vi "Img Update Basic Point.vi"(8 "error in (no error)":errorcluster, 11 "LF2R IDE in":refnum<class "Main Panel.lvclass">) -> (0 "error out":errorcluster, 3 "LF2R IDE out":refnum<class "Main Panel.lvclass">)   [LabVIEW 2018, in "Main Panel.lvlib" / "Main Panel.lvclass"]
uses:
  Main Panel.lvclass
  Main Panel.lvclass/Main Panel.ctl
  Image/Image Process.lvclass
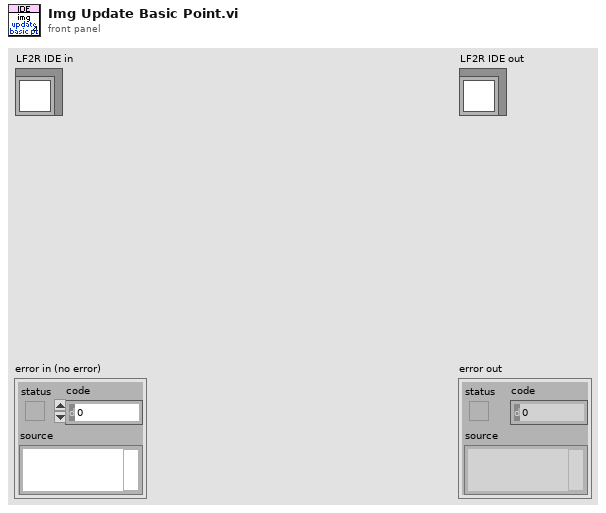
[diagram p1: front panel]
types:
  T1 = typedef "IMAQ Image.ctl" = refnum<image>
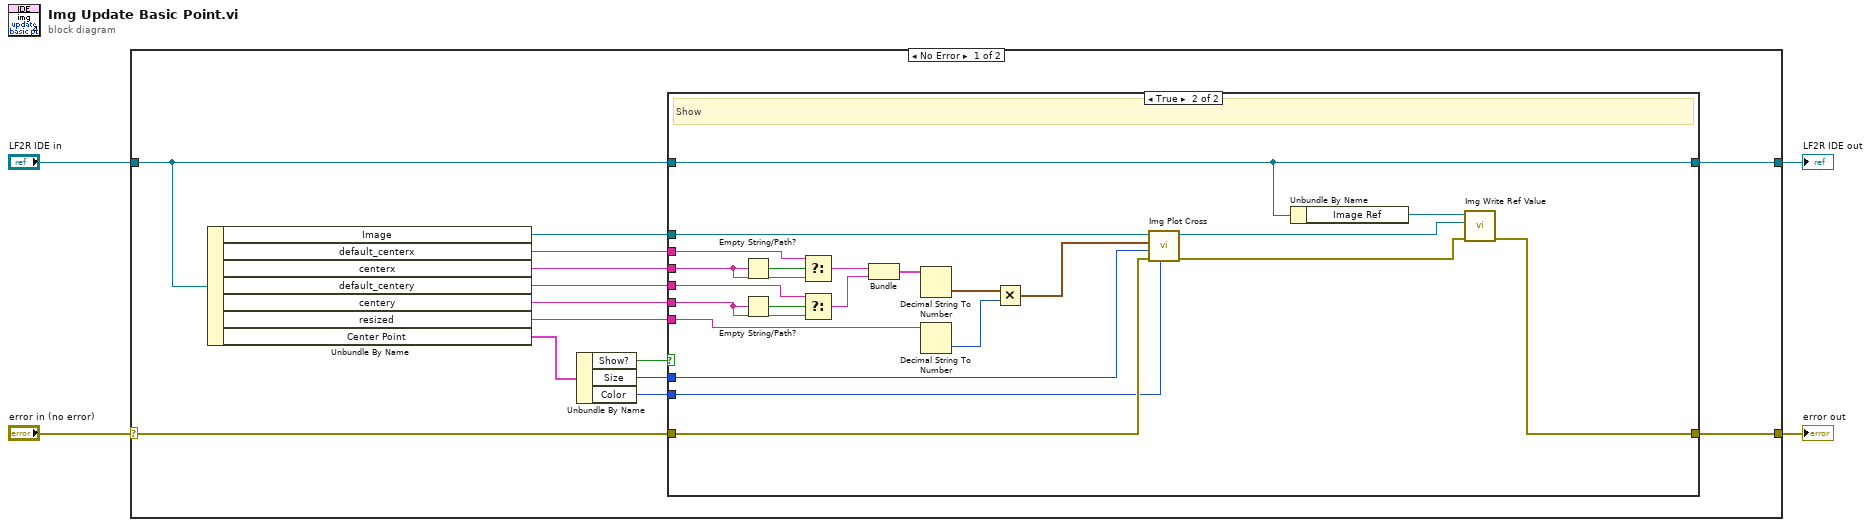
[diagram p0: block diagram]
diagram:
  n1 = case shown="No Error" "error in (no error)" {
    selector: "error in (no error)" -> [w10 w44]
    tunnel: [w17 w44] -> w3
    tunnel: [w8 w43] -> w1
    tunnel: "LF2R IDE in" -> [w18 w43]
    frame No Error {
      n2 = Unbundle By Name(w18) -> ("Image"=w11:T1, "default_centerx"=w15:string, "centerx"=w14:string, "default_centery"=w13:string, "centery"=w12:string, "resized"=w16:string, "Center Point"=w9:cluster{"Size":i32, "Color":u32, "Show?":bool})
      n3 = Unbundle By Name(w9) -> ("Show?"=w7:bool, "Size"=w6:i32, "Color"=w5:u32)
      n4 = case shown="True" w7 {
        tunnel: w18 -> [w20 w23]
        tunnel: [w19 w41] -> w17
        tunnel: w16 -> [_ w40]
        tunnel: w15 -> [_ w36]
        tunnel: w14 -> [_ w35]
        tunnel: w13 -> [_ w33]
        tunnel: w12 -> [_ w32]
        tunnel: w11 -> [_ w28]
        tunnel: w10 -> [w19 w26]
        tunnel: [w20 w23] -> w8
        tunnel: w6 -> [_ w22]
        tunnel: w5 -> [_ w21]
        frame False {
          # "Skip"
        }
        frame True {
          # "Show"
          n5 = Empty String/Path?(string/path=w35) -> (empty?=w37:bool)
          n6 = Empty String/Path?(string/path=w32) -> (empty?=w34:bool)
          n7 = Select(t=w36, s=w37, f=w35) -> (s? t:f=w31:string)
          n8 = Select(t=w33, s=w34, f=w32) -> (s? t:f=w30:string)
          n9 = Bundle("centerx"=w31, "centery"=w30) -> (w29:cluster{"centerx":string, "centery":string})  [unwired: 1 in]
          n10 = Decimal String To Number(string=w29) -> (number=w39:cluster{"centerx":i32, "centery":i32})  [unwired: 2 in, 1 out]
          n11 = Decimal String To Number(string=w40) -> (number=w38:i32)  [unwired: 2 in, 1 out]
          n12 = Multiply(x=w39, y=w38) -> (x*y=w27:cluster{"centerx":i32, "centery":i32})
          n13 = call "Img Plot Cross.vi"("Color"=w21, "error in (no error)"=w26, "size"=w22, "position"=w27, "Image In"=w28) -> ("error out"=w25:errorcluster, "Image Out"=w24:T1)  [unwired: 5 in]
          n14 = Unbundle By Name(w23) -> ("Image Ref"=w42:refnum<vi>)
          n15 = call "Img Write Ref Value.vi"("error in (no error)"=w25, "Image"=w24, "Image Ref"=w42) -> ("error out"=w41:errorcluster)  [unwired: 8 in]
        }
      }
    }
    frame Error {
    }
  }
  "error out" <- w3
  "LF2R IDE out" <- w1
